vi "Proyecto Autotronica.vi"() -> ()   [LabVIEW 2025]
uses:
  <vilib>/MakerHub/LINX/Private/Type Defs/LINX Ref.ctl
  <vilib>/MakerHub/LINX/Private/Type Defs/Platform.ctl
  <vilib>/MakerHub/LINX/Private/Type Defs/Interface.ctl
  <vilib>/MakerHub/LINX/Private/Device/Type Defs/LINX Device Config.ctl
  <vilib>/MakerHub/LINX/Private/Device/Type Defs/TCP Config.ctl
  <vilib>/MakerHub/LINX/Private/Device/Type Defs/Channels.ctl
  <vilib>/MakerHub/LINX/Public/Peripherals/Digital/Digital Read 1 Chan.vi
  <vilib>/MakerHub/LINX/Public/Peripherals/Analog/Analog Read 1 Chan.vi
  <vilib>/MakerHub/LINX/Public/Peripherals/Digital/Digital Read N Chans.vi
  <vilib>/MakerHub/LINX/Public/Peripherals/Analog/Analog Read N Chans.vi
  <vilib>/MakerHub/LINX/Private/Local IO/LinxDigitalRead.vi
  <vilib>/MakerHub/LINX/Public/Utilities/Check Channel.vi
  <vilib>/MakerHub/LINX/Private/Local IO/LinxAnalogRead.vi
  <vilib>/MakerHub/LINX/Public/Utilities/Open Serial.vi
  <vilib>/MakerHub/LINX/Private/Utilties/Generate Error.vi
  <vilib>/express/express shared/transition.llb/Dynamic To Waveform Array.vi
  <vilib>/express/express signal manip/GetorSetDDTAttributes/Set DDT Attributes/SetT0.vi
  <vilib>/express/express shared/transition.llb/Waveform Array To Dynamic.vi
  <vilib>/express/express arith-compare/Formula/XNode/ExpressFormulaBlockNode.xnode
  <vilib>/express/express signal manip/GetorSetDDTAttributes/Set DDT Attributes/Set DDT Properties.xnode
  <vilib>/MakerHub/LINX/LMH-LINX.lvlib
  <vilib>/MakerHub/LINX/Private/Device/Device.lvlib
panel:
  out "Waveform Chart":dbl(graph)
  out "Presion de frenado":dbl(knob) scale=0.0..50.0
  out "Batería":dbl(slide) scale=0.0..100.0
  out "Celsius":dbl(slide) scale=0.0..300.0
  out "Kelvin":dbl(slide) scale=0.0..300.0
  out "Fahrenheit":dbl(slide) scale=0.0..300.0
  out "RPMs":dbl(knob) scale=0.0..5000.0
  in  "Serial Port":refnum<visa-resource-name>="N/A"
  in  "stop":bool
  # "Temperaturas"
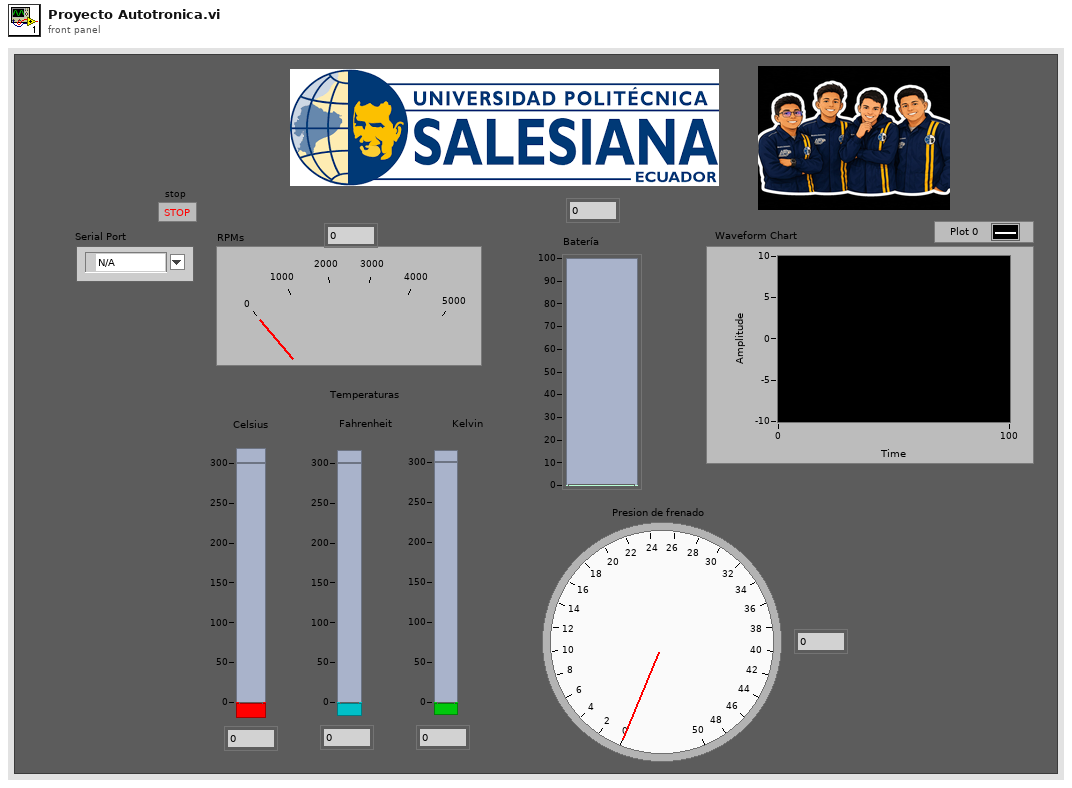
[diagram p1: front panel]
types:
  T1 = typedef "LMH-LINX.lvlib/LINX Ref.ctl" = cluster{"IO":T2, "Interface":T3, "LINX Device Config":T4}
  T2 = typedef "LMH-LINX.lvlib/Platform.ctl" = enum16{"Remote", "Local"}
  T3 = typedef "LMH-LINX.lvlib/Interface.ctl" = enum16{"Serial", "TCP"}
  T4 = typedef "LMH-LINX.lvlib/Device.lvlib/LINX Device Config.ctl" = cluster{"Interface":T3, "COM Port":refnum<visa-resource-name>, "TCP Configuration":T5, "Device Family":u8, "Device ID":u8, "Device Name":string, "TCP Ref":refnum<k5>, "Channels":T6}
  T5 = typedef "LMH-LINX.lvlib/Device.lvlib/TCP Config.ctl" = cluster{"IP Address":string, "Port":u16}
  T6 = typedef "LMH-LINX.lvlib/Channels.ctl" = cluster{"DI":u8[], "DO":u8[], "AI":u8[], "AO":u8[], "PWM":u8[], "QE":u8[], "UART":u8[], "I2C 2":u8[], "SPI":u8[], "CAN":u8[], "Servo":u8[], "AI Ref (V)":dbl, "AI Resolution (Bits)":u8, "AO Ref (V)":dbl, "AO Resolution (Bits)":u8}
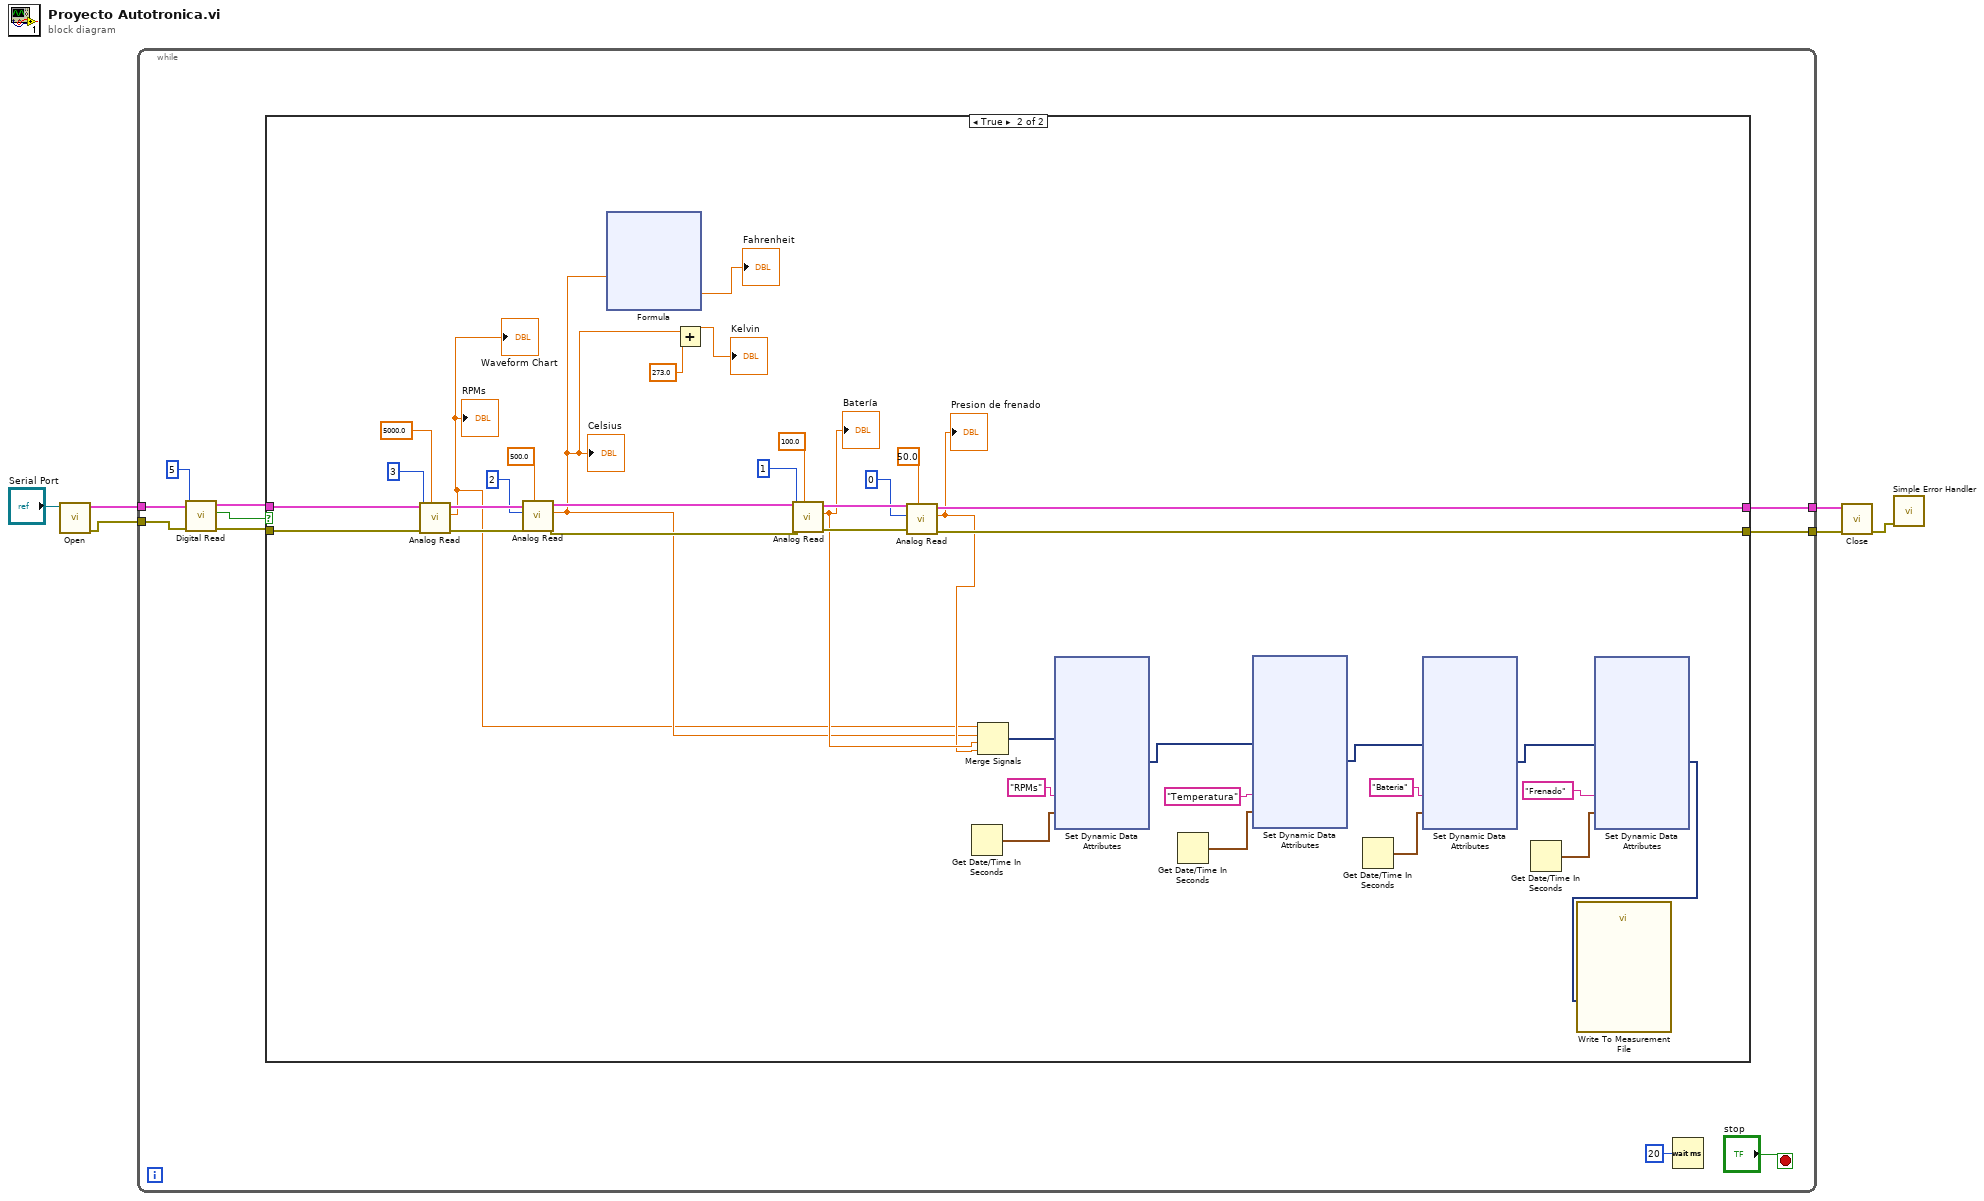
[diagram p0: block diagram]
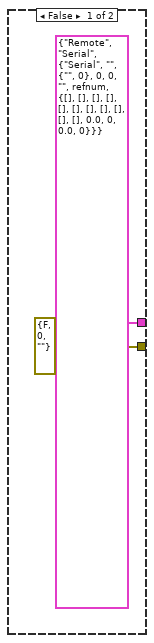
[diagram p2: hidden frame]
diagram:
  n1 = call-poly <vilib>:"Open.vi"("Serial Port"="Serial Port") -> ("Error Out"=w5:errorcluster, "LINX Resource"=w6:T1)  [unwired: 8 in, 1 out]
  n2 = while {
    tunnel: w6 -> [w14]
    tunnel: w5 -> [w13]
    tunnel: [w8] -> w2
    tunnel: [w7] -> w1
    stop <- "stop" stop-if-true
    n3 = call-poly <vilib>:"Digital Read.vi"("Error In"=w13, "DI Channel"=u8 5, "LINX Resource"=w14) -> ("Error Out"=w11:errorcluster, "DI Value"=w10:bool, "LINX Resource"=w12:T1)  [unwired: 6 in]
    n4 = case shown="True" w10 {
      tunnel: w12 -> [_ w56]
      tunnel: w11 -> [_ w53]
      tunnel: [errorcluster {"status"=FALSE, "code"=0, "source"=""} ("Error Out") w41] -> w8
      tunnel: [T1 {"IO"=enum."Remote", "Interface"=enum."Serial", "LINX Device Config"={"Interface"=enum."Serial", "COM Port"="", "TCP Configuration"={"IP Address"="", "Port"=0}, "Device Family"=0, "Device ID"=0, "Device Name"="", "TCP Ref"=refnum, "Channels"={"DI"=[], "DO"=[], "AI"=[], "AO"=[], "PWM"=[], "QE"=[], "UART"=[], "I2C 2"=[], "SPI"=[], "CAN"=[], "Servo"=[], "AI Ref (V)"=0.0, "AI Resolution (Bits)"=0, "AO Ref (V)"=0.0, "AO Resolution (Bits)"=0}}} ("LINX Resource") w39] -> w7
      frame False {
      }
      frame True {
        n5 = call-poly <vilib>:"Analog Read.vi"("Analog Ref Override (V)"=5000.0, "Error In"=w53, "Analog Channel"=u8 3, "LINX Resource"=w56) -> ("Error Out"=w52:errorcluster, "Voltage"=w19:dbl, "LINX Resource"=w55:T1)  [unwired: 4 in, 1 out]
        "RPMs" <- w19
        "Waveform Chart" <- w19
        n6 = call-poly <vilib>:"Analog Read.vi"("Analog Ref Override (V)"=500.0, "Error In"=w52, "Analog Channel"=u8 2, "LINX Resource"=w55) -> ("Error Out"=w51:errorcluster, "Voltage"=w27:dbl, "LINX Resource"=w54:T1)  [unwired: 4 in, 1 out]
        "Celsius" <- w27
        n7 = xnode "Formula"("X1"=w27) -> ("Result"=→"Fahrenheit":dbl)  [unwired: 1 in, 1 out]
        n8 = Add(x=w27, y=273.0) -> (x+y=→"Kelvin":dbl)
        n9 = call-poly <vilib>:"Analog Read.vi"("Analog Ref Override (V)"=100.0, "Error In"=w51, "Analog Channel"=u8 1, "LINX Resource"=w54) -> ("Error Out"=w42:errorcluster, "Voltage"=w29:dbl, "LINX Resource"=w40:T1)  [unwired: 4 in, 1 out]
        "Batería" <- w29
        n10 = call-poly <vilib>:"Analog Read.vi"("Analog Ref Override (V)"=50.0, "Error In"=w42, "Analog Channel"=u8 0, "LINX Resource"=w40) -> ("Error Out"=w41:errorcluster, "Voltage"=w28:dbl, "LINX Resource"=w39:T1)  [unwired: 4 in, 1 out]
        "Presion de frenado" <- w28
        n11 = Get Date/Time In Seconds() -> (seconds since 1Jan1904=w26:timestamp)
        n12 = Merge Signals(w19, w27, w29, w28) -> (w38:dynamicdata)
        n13 = xnode "Set Dynamic Data Attributes"("Signals In"=w38, "Signal Name"="RPMs", "Timestamp"=w26) -> ("Signals Out"=w36:dynamicdata)  [unwired: 2 in, 1 out]
        n14 = Get Date/Time In Seconds() -> (seconds since 1Jan1904=w25:timestamp)
        n15 = xnode "Set Dynamic Data Attributes"("Signals In"=w36, "Signal Name"="Temperatura", "Timestamp"=w25) -> ("Signals Out"=w35:dynamicdata)  [unwired: 2 in, 1 out]
        n16 = Get Date/Time In Seconds() -> (seconds since 1Jan1904=w24:timestamp)
        n17 = xnode "Set Dynamic Data Attributes"("Signals In"=w35, "Signal Name"="Bateria", "Timestamp"=w24) -> ("Signals Out"=w34:dynamicdata)  [unwired: 2 in, 1 out]
        n18 = Get Date/Time In Seconds() -> (seconds since 1Jan1904=w23:timestamp)
        n19 = xnode "Set Dynamic Data Attributes"("Signals In"=w34, "Signal Name"="Frenado", "Timestamp"=w23) -> ("Signals Out"=w33:dynamicdata)  [unwired: 2 in, 1 out]
        n20 = call "Write To Measurement File"("Signals"=w33) -> ()  [unwired: 16 in, 3 out]
      }
    }
    n21 = Wait (ms)(milliseconds to wait=u32 20) -> ()  [unwired: 1 out]
  }
  n22 = call <vilib>:"Close.vi"("Error In"=w2, "LINX Resource"=w1) -> ("Error Out"=w4:errorcluster)  [unwired: 9 in]
  n23 = call <vilib>:"Simple Error Handler.vi"("error in (no error)"=w4) -> ()  [unwired: 4 in, 5 out]
